vi "Tell.vi"(10 "Msg":refnum<class "Msg.lvclass">, 11 "Transport in":refnum<class "Transport.lvclass">) -> (0 "Error out":errorcluster)   [LabVIEW 2025, in "jettl.lvlib" / "Transport.lvlib" / "Transport.lvclass"]
uses:
  Transport.lvclass
  Msg/Msg.lvclass
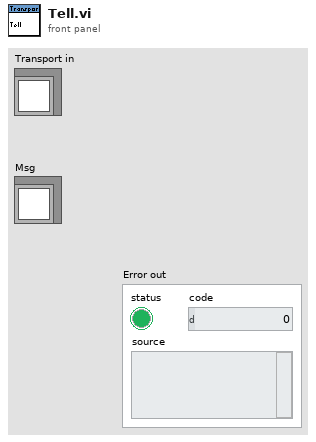
[diagram p1: front panel]
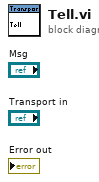
[diagram p0: block diagram]
diagram:
